vi "Read Y Component.vi"(8 "error in (no error)":errorcluster, 10 "component":T1=32 items=["Magnitude^2"=37, "Magnitude"=32, "Phase"=33, "Real"=34, "Imaginary"=35], 11 "Y (Complex) (1Ch) in":refnum<class "Y (Complex) (1 Ch).lvclass">) -> (0 "error out":errorcluster, 2 "Y":dbl[](array[numeric]), 3 "Y (Complex) (1Ch) out":refnum<class "Y (Complex) (1 Ch).lvclass">)   [LabVIEW 2017, in "Y (Complex) (1 Ch).lvclass"]
uses:
  <vilib>/addons/_NISVFA/_Shared subVIs/Data Objects/Y (Complex) (DBL)/Y (Complex) (1 Ch).lvclass
  <vilib>/addons/_NISVFA/_Shared subVIs/Controls/NI Spectrum Component.ctl
  <vilib>/addons/_NISVFA/_Shared subVIs/Data Objects/Y (Complex) (DBL)/Y (Complex) (1 Ch).lvclass/Y (Complex) (1 Ch).ctl
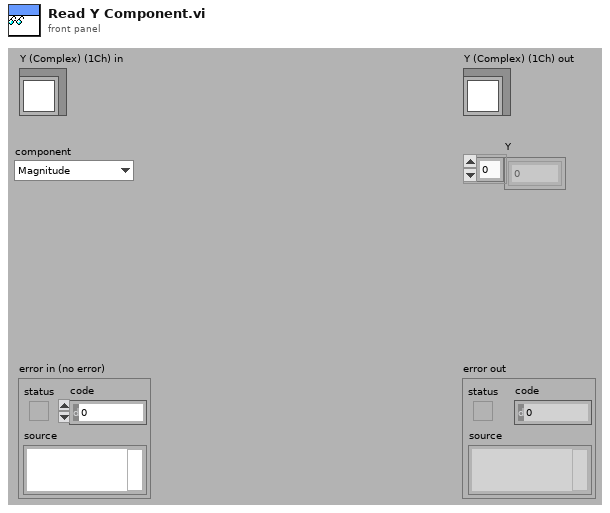
[diagram p1: front panel]
types:
  T1 = typedef "NI Spectrum Component.ctl" = u16
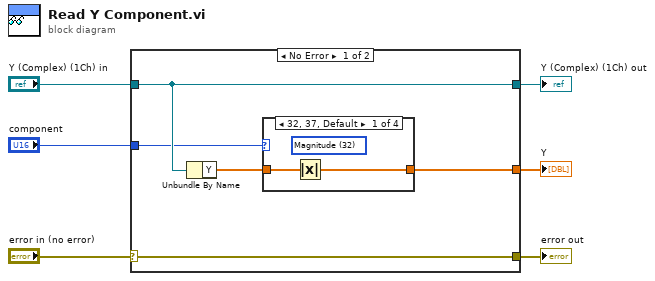
[diagram p0: block diagram]
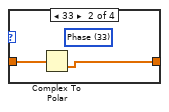
[diagram p2: hidden frame]
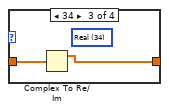
[diagram p3: hidden frame]
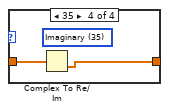
[diagram p4: hidden frame]
diagram:
  n1 = case shown="No Error" "error in (no error)" {
    selector: "error in (no error)" -> [w11 w20]
    tunnel: [w11 w20] -> w5
    tunnel: [w10 w21] -> w3
    tunnel: "Y (Complex) (1Ch) in" -> [w10 w21]
    tunnel: [w7 _] -> w2
    tunnel: "component" -> [w9 _]
    frame No Error {
      n2 = Unbundle By Name(w10) -> ("Y"=w8:cdb[])
      n3 = case shown="32, 37, Default" w9 {
        tunnel: w8 -> [w13 w15 w17 w19]
        tunnel: [w12 w14 w16 w18] -> w7
        frame 32, 37, Default {
          (unwired) T1 32 items=["Magnitude"=32, "Phase"=33, "Real"=34, "Imaginary"=35, "Coherence"=36, "Unknown"=99] ("component")
          n4 = Absolute Value(x=w13) -> (abs(x)=w12:dbl[])
        }
        frame 33 {
          (unwired) T1 33 items=["Magnitude"=32, "Phase"=33, "Real"=34, "Imaginary"=35, "Coherence"=36, "Unknown"=99] ("component")
          n5 = Complex To Polar(r * e^(i*theta)=w15) -> (theta=w14:dbl[])  [unwired: 1 out]
        }
        frame 34 {
          (unwired) T1 34 items=["Magnitude"=32, "Phase"=33, "Real"=34, "Imaginary"=35, "Coherence"=36, "Unknown"=99] ("component")
          n6 = Complex To Re/Im(x + iy=w17) -> (x=w16:dbl[])  [unwired: 1 out]
        }
        frame 35 {
          (unwired) T1 35 items=["Magnitude"=32, "Phase"=33, "Real"=34, "Imaginary"=35, "Coherence"=36, "Unknown"=99] ("component")
          n7 = Complex To Re/Im(x + iy=w19) -> (y=w18:dbl[])  [unwired: 1 out]
        }
      }
    }
    frame Error {
    }
  }
  "error out" <- w5
  "Y (Complex) (1Ch) out" <- w3
  "Y" <- w2
